vi "GameOfLife.vi"() -> ()   [LabVIEW 2020]
uses:
  Ctrls/ElementalCell.ctl
panel:
  in  "Main Board":T1[][](array[typedef])
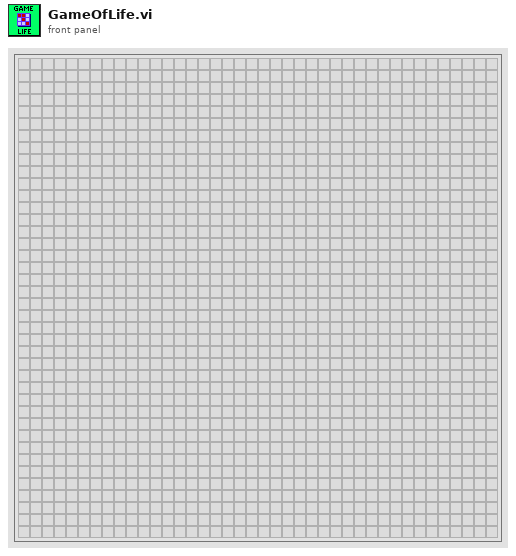
[diagram p1: front panel]
types:
  T1 = typedef "ElementalCell.ctl" = bool
  T2 = typedef "MainData.ctl" = cluster{"Size":i32, "Live rule":i32[], "Dead rule":i32[]}
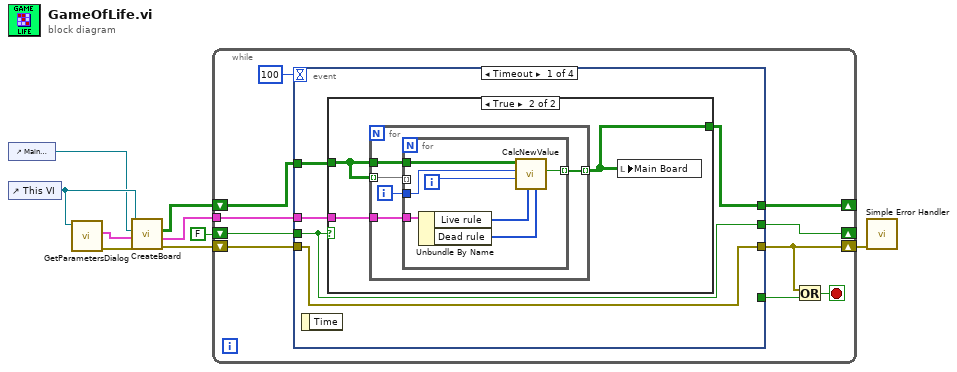
[diagram p0: block diagram]
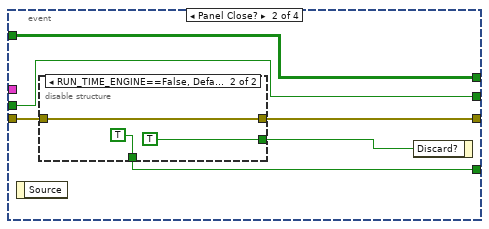
[diagram p3: hidden frame]
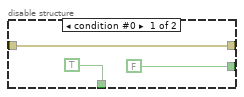
[diagram p4: hidden frame]
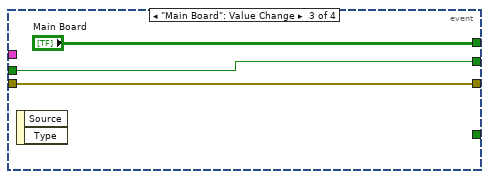
[diagram p5: hidden frame]
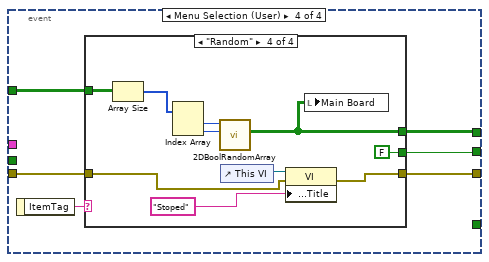
[diagram p6: hidden frame]
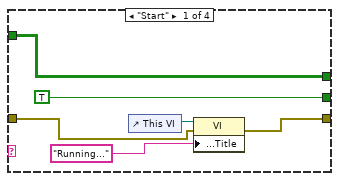
[diagram p7: hidden frame]
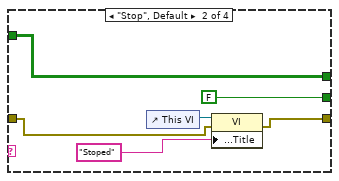
[diagram p8: hidden frame]
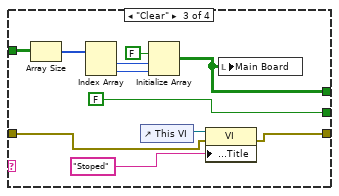
[diagram p9: hidden frame]
diagram:
  n1 = control-ref of="Main Board"() -> (w1:refnum<vi>)
  n2 = control-ref of="This VI"() -> (w5:refnum<vi>)
  n3 = call "GetParametersDialog.vi"("Main VI Ref"=w5) -> ("Error Out"=w4:errorcluster, "MainData"=w3:T2)  [unwired: 7 in]
  n4 = call "CreateBoard.vi"("Error In"=w4, "Param In"=w3, "Arr Ref"=w1, "Main VI Ref"=w5) -> ("Error Out"=w9:errorcluster, "Param Out"=w2:T2, "Main Board"=w7:T1[][])  [unwired: 5 in]
  n5 = while {
    shift-right: [w12] -> w8
    shift-left: w9 -> [w18]
    shift-right: [w14] -> _
    shift-left: w7 -> [w17]
    shift-right: [w15] -> _
    shift-left: FALSE -> [w16]
    tunnel: w2 -> [w10]
    stop <- w13 stop-if-true
    n6 = event shown="[0] Timeout" {
      selector: _ -> [_ _ _ _]
      dyn-events: _ -> [_ _ _ _]
      timeout: 100 -> [_ _ _ _]
      tunnel: w18 -> [w24 w44 w53 w60]
      tunnel: [w24 w43 w53 w56] -> w12
      tunnel: w17 -> [w23 w41 _ w59]
      tunnel: w16 -> [w22 w42 w54 _]
      tunnel: [w22 w42 w54 w57] -> w15
      tunnel: [w21 w41 "Main Board" w58] -> w14
      tunnel: [_ w45 _ _] -> w11
      tunnel: w10 -> [w20 _ _ _]
      event Timeout {
        n7 = event-data() -> ()  [unwired: 1 in, 1 out]
        n8 = case shown="True" w22 {
          tunnel: w23 -> [w25 w27]
          tunnel: [w25 w28] -> w21
          tunnel: w20 -> [_ w26]
          frame False {
          }
          frame True {
            n9 = for {
              tunnel: w27 -> [w32] mode=indexing
              tunnel: w27 -> [w31]
              tunnel: [w30] -> w28 mode=indexing
              tunnel: w26 -> [w29]
              i -> [w33]
              n10 = for {
                tunnel: w33 -> [w40]
                tunnel: w32 -> [_] mode=indexing
                tunnel: w31 -> [w38]
                tunnel: [w37] -> w30 mode=indexing
                tunnel: w29 -> [w36]
                i -> [w39]
                n11 = Unbundle By Name(w36) -> ("Live rule"=w35:i32[], "Dead rule"=w34:i32[])
                n12 = call "CalcNewValue.vi"("Dead rule"=w34, "Live rule"=w35, "j"=w39, "i"=w40, "Main Board"=w38) -> ("New value"=w37:T1)  [unwired: 6 in]
              }
            }
            n13 = local write "Main Board"(w28) -> ()
          }
        }
      }
      event Panel Close? {
        n14 = event-data() -> ()  [unwired: 1 in, 1 out]
        n15 = disable-structure shown="RUN_TIME_ENGINE==False, Default" {
          disable-tunnel: [FALSE TRUE] -> w46
          disable-tunnel: [TRUE TRUE] -> w45
          disable-tunnel: w44 -> [w48 w50]
          disable-tunnel: [w48 w50] -> w43
          frame condition #0 {
          }
          frame condition #1 (active) {
          }
        }
        n16 = event-data("Discard?"=w46) -> ()  [unwired: 1 in, 1 out]
      }
      event "Main Board": Value Change {
        n17 = event-data() -> ()  [unwired: 1 in, 2 out]
      }
      event Menu Selection (User) {
        n18 = event-data() -> ("ItemTag"=w61:string)  [unwired: 1 in]
        n19 = case shown="\"Random\"" w61 {
          tunnel: w60 -> [w64 w69 w75 w86]
          tunnel: w59 -> [w67 w72 w82 w93]
          tunnel: [w67 w72 w78 w89] -> w58
          tunnel: [TRUE FALSE FALSE FALSE] -> w57
          tunnel: [w63 w68 w74 w85] -> w56
          frame "Start" {
            n20 = control-ref of="This VI"() -> (w65:refnum<vi>)
            n21 = property class="VI"(reference=w65, error in=w64, "Front Panel.Title"="Running..." ("Front Panel Window:Title")) -> (error out=w63:errorcluster)  [unwired: 1 out]
          }
          frame "Stop", Default {
            n22 = control-ref of="This VI"() -> (w71:refnum<vi>)
            n23 = property class="VI"(reference=w71, error in=w69, "Front Panel.Title"="Stoped" ("Front Panel Window:Title")) -> (error out=w68:errorcluster)  [unwired: 1 out]
          }
          frame "Clear" {
            n24 = Array Size(array=w82) -> (size(s)=w81:i32[])
            n25 = Index Array(array=w81) -> (element #1=w80:i32, element #2=w79:i32)  [unwired: 2 in]
            n26 = control-ref of="This VI"() -> (w77:refnum<vi>)
            n27 = Initialize Array(T1 FALSE ("Boolean"), w80, w79) -> (w78:T1[][])
            n28 = property class="VI"(reference=w77, error in=w75, "Front Panel.Title"="Stoped" ("Front Panel Window:Title")) -> (error out=w74:errorcluster)  [unwired: 1 out]
            n29 = local write "Main Board"(w78) -> ()
          }
          frame "Random" {
            n30 = Array Size(array=w93) -> (size(s)=w92:i32[])
            n31 = Index Array(array=w92) -> (element #1=w91:i32, element #2=w90:i32)  [unwired: 2 in]
            n32 = call "2DBoolRandomArray.vi"("j"=w90, "i"=w91) -> ("Main Board"=w89:T1[][])  [unwired: 9 in]
            n33 = control-ref of="This VI"() -> (w88:refnum<vi>)
            n34 = property class="VI"(reference=w88, error in=w86, "Front Panel.Title"="Stoped" ("Front Panel Window:Title")) -> (error out=w85:errorcluster)  [unwired: 1 out]
            n35 = local write "Main Board"(w89) -> ()
          }
        }
      }
    }
    n36 = Or(x=w12, y=w11) -> (x .or. y?=w13:bool)
  }
  n37 = call <vilib>:"Simple Error Handler.vi"("error in (no error)"=w8) -> ()  [unwired: 4 in, 5 out]
